vi "LVClass_SlopesPostProcessList AddProcessor_NeighboorExtension.vi"(0 "SlopesPostProcessorList in":refnum<class "SlopesPostProcessorList.lvclass">, 5 "Position":i32, 11 "error in (no error)":errorcluster) -> (4 "SlopesPostProcessorList out":refnum<class "SlopesPostProcessorList.lvclass">, 15 "error out":errorcluster)   [LabVIEW 2020, in "SlopesPostProcessorList.lvclass"]
doc: "Insert a NeighborExtension processor.\n\n--------------------------------------------------------------------------------\n\n<B>SlopesPostProcessorListIn </B> : SlopesPostProcessorList object.\n<B>SlopesPostProcessorListOut </B> : SlopesPostProcessorList object.\n<B>position </B> : Position of the processor in the SlopesPostProcessorList.\n<B>ErrorIn </B> : Error\n<B>ErrorOut </B> : Error\n\n--------------------------------------------------------------------------------"
uses:
  SlopesPostProcessorList.lvclass
  SlopesPostProcessorList.lvclass/SlopesPostProcessorList.ctl
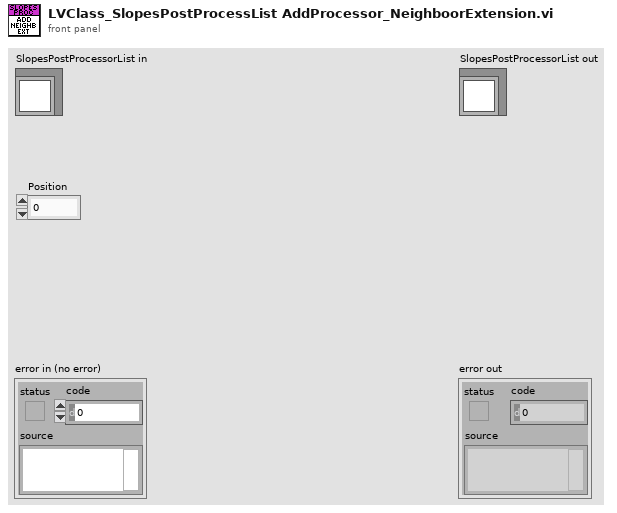
[diagram p1: front panel]
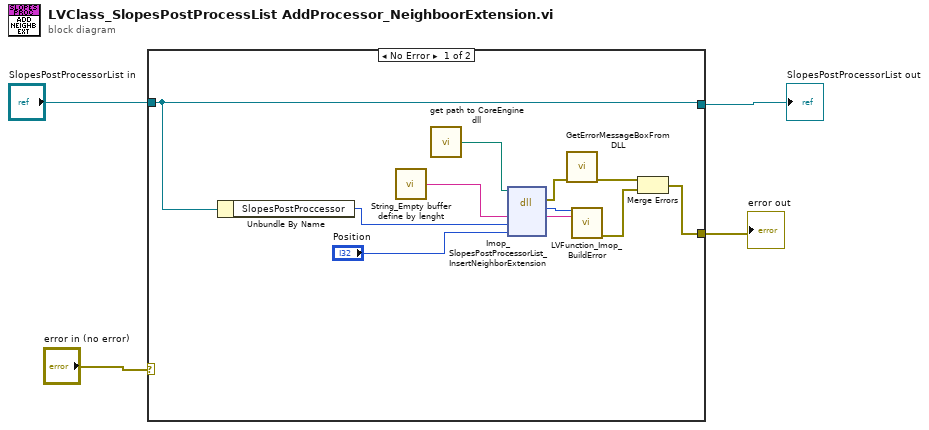
[diagram p0: block diagram]
diagram:
  n1 = case shown="No Error" "error in (no error)" {
    selector: "error in (no error)" -> [_ w16]
    tunnel: "SlopesPostProcessorList in" -> [w9 w17]
    tunnel: [w9 w17] -> w2
    tunnel: [w5 w16] -> w1
    frame No Error {
      n2 = Unbundle By Name(w9) -> ("SlopesPostProccessor"=w8:i32)
      n3 = call "String_Empty buffer define by lenght.vi"() -> ("Empty buffer"=w15:string)  [unwired: 1 in]
      n4 = call "get path to CoreEngine dll.vi"() -> ("path to c_interface_vc100.dll"=w12:path)  [unwired: 12 in, 3 out]
      n5 = dll-call lib="D:/soft/HASO_v3/SVN_trunk/ImOpCoreEngine4_LV2011/DLLs/c_interface_vc100.dll" fn="Imop_SlopesPostProcessorList_InsertNeighborExtension"(path in=w12, "message"=w15, "objet"=w8, "Position"="Position") -> (error out=w11:errorcluster, "return type"=w13:i32, "message"=w14:string)  [unwired: 4 in, 1 out]
      n6 = call "GetErrorMessageBoxFromDLL.vi"("error IN"=w11) -> ("error OUT"=w7:errorcluster)  [unwired: 10 in]
      n7 = call "LVFunction_Imop_BuildError.vi"("code"=w13, "String to Prepend to source (\"\")"=w14) -> ("error out"=w6:errorcluster)  [unwired: 13 in]
      n8 = Merge Errors(w7, w6) -> (w5:errorcluster)
    }
    frame Error {
    }
  }
  "error out" <- w1
  "SlopesPostProcessorList out" <- w2
